vi "Queue Basics.vi"() -> ()   [LabVIEW 2012]
doc: "该范例演示了“获取队列引用”的使用方法，以及不同设置对队列操作的影响。通过队列在元素入队列（产生数据）和元素出队列（消费数据）之间传递数据。如两个循环的速度相同，队列将不会被填满。\n\n如元素入队列循环的速度大于元素出队列的速度，队列将被填满。元素入队列循环必须等待元素出队列循环移出队列中的元素。如元素入队列循环的速度小于元素出队列的速度，队列将被清空。元素出队列循环必须等待元素入队列循环填充队列中的元素。"
panel:
  out "Last Element Removed":dbl caption="最后删除的元素" format="%0.2f"
  in  "Enqueue Speed":bool caption="入队列速度"
  in  "Dequeue Speed":bool caption="出队列速度"
  out "Waveform Chart":cluster{"Last Element Inserted":dbl, dbl}(graph) caption="波形图表"
  out "Elements in Queue":i32(slide) caption="队列中的元素" scale=0.0..50.0 scale format="%0.0f"
  in  "stop":bool caption="停止"
  in  "Queue Size":i32=50 caption="队列大小"
  out "Last Element Inserted":dbl caption="最后插入的元素" format="%0.2f"
  # "操作步骤：\n1.设置要使用的队列大小。\n2.运行VI。\n3.调整“入队列速度”输入控件和“出队列速度”输入控件的值，查看队列显示控件中的元素和波形图表中曲线的改变。"
  # "最快(100ms)\n最慢(500ms)"
  # "最快(100ms)\n最慢(500ms)"
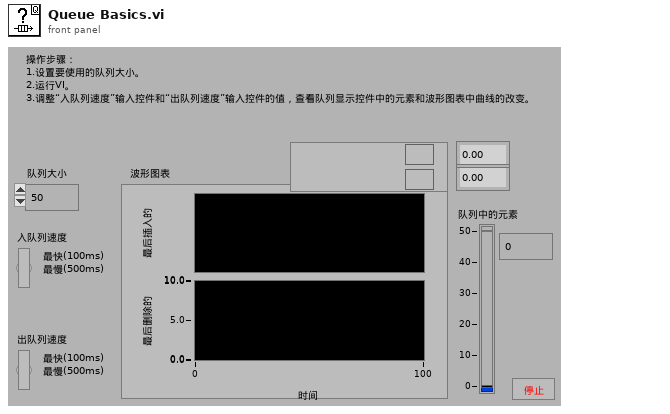
[diagram p1: front panel]
types:
  T1 = cluster{"Last Element Inserted":dbl, "Last Element Removed":dbl}
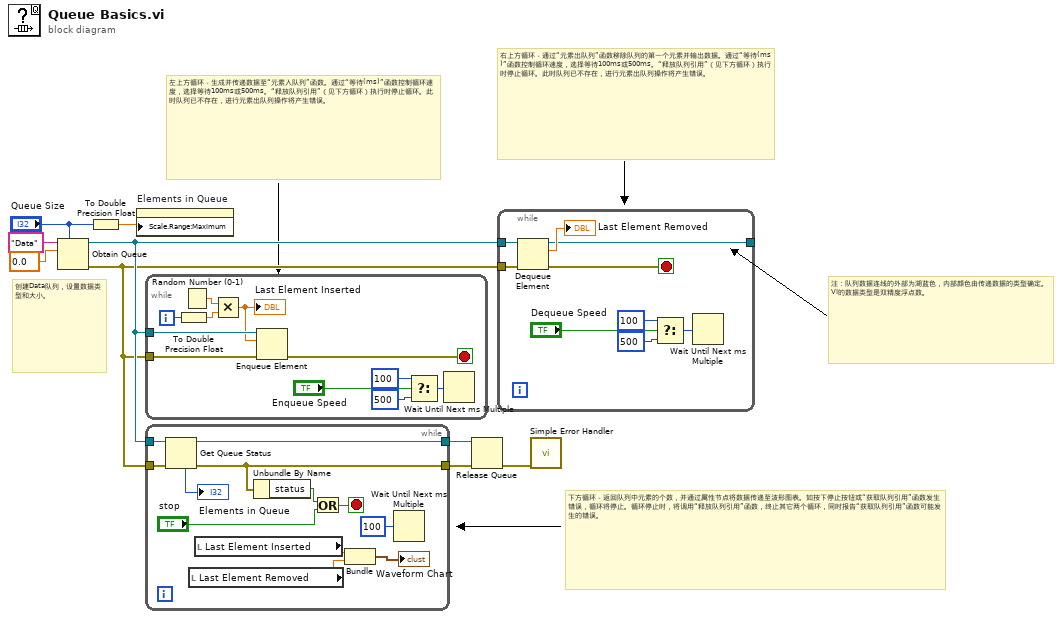
[diagram p0: block diagram]
diagram:
  # "右上方循环－通过“元素出队列”函数移除队列的第一个元素并输出数据。通过“等待(ms)”函数控制循环速度，选择等待100ms或500ms。“释放队列引用”（见下方循环）执行时停止循环。此时队列已不存在，进行元素出队列操作将产生错误。"
  # "注：队列数据连线的外部为湖蓝色，内部颜色由传递数据的类型确定。VI的数据类型是双精度浮点数。"
  # "下方循环－返回队列中元素的个数，并通过属性节点将数据传递至波形图表。如按下停止按钮或“获取队列引用”函数发生错误，循环将停止。循环停止时，将调用“释放队列引用”函数，终止其它两个循环，同时报告“获取队列引用”函数可能发生的错误。"
  # "左上方循环－生成并传递数据至“元素入队列”函数。通过“等待(ms)”函数控制循环速度，选择等待100ms或500ms。“释放队列引用”（见下方循环）执行时停止循环。此时队列已不存在，进行元素出队列操作将产生错误。"
  # "创建Data队列，设置数据类型和大小。"
  n1 = Obtain Queue(max queue size (-1, unlimited)="Queue Size", name (unnamed)="Data", element data type=0.0) -> (queue out=w9:refnum<queue>, error out=w4:errorcluster)  [unwired: 2 in, 1 out]
  n2 = To Double Precision Float(number="Queue Size") -> (double precision float=w8:dbl)
  n3 = property on="Elements in Queue" class="Slide (严格)"("Scale.Range:Maximum"=w8) -> ()  [unwired: 2 in, 2 out]
  n4 = while {
    tunnel: w9 -> [w20]
    tunnel: w4 -> [w11]
    i -> [w18]
    stop <- w10 stop-if-true
    n5 = To Double Precision Float(number=w18) -> (double precision float=w17:dbl)
    n6 = Random Number (0-1)() -> (number: 0 to 1=w19:dbl)
    n7 = Multiply(x=w19, y=w17) -> (x*y=w16:dbl)
    "Last Element Inserted" <- w16
    n8 = Enqueue Element(queue=w20, element=w16, error in (no error)=w11) -> (error out=w10:errorcluster)  [unwired: 3 out]
    n9 = Select(t=u32 100, s="Enqueue Speed", f=u32 500) -> (s? t:f=w12:u32)
    n10 = Wait Until Next ms Multiple(millisecond multiple=w12) -> ()  [unwired: 1 out]
  }
  n11 = while {
    tunnel: w9 -> [w32]
    tunnel: [w21] -> w3
    tunnel: w4 -> [w25]
    tunnel: [w22] -> w2
    stop <- w28 stop-if-true
    n12 = Get Queue Status(queue=w32, error in (no error)=w25) -> (queue out=w22:refnum<queue>, error out=w21:errorcluster, # elements in queue=→"Elements in Queue":i32)  [unwired: 6 out]
    n13 = local read "Last Element Removed"() -> (w23:dbl)
    n14 = local read "Last Element Inserted"() -> (w24:dbl)
    n15 = Unbundle By Name(w21) -> ("status"=w27:bool)
    n16 = Or(x=w27, y="stop") -> (x .or. y?=w28:bool)
    n17 = Bundle("Last Element Inserted"=w24, "Last Element Removed"=w23) -> (→"Waveform Chart":T1)  [unwired: 1 out]
    n18 = Wait Until Next ms Multiple(millisecond multiple=u32 100 ("milliseconds to wait")) -> ()  [unwired: 1 out]
  }
  n19 = Release Queue(queue=w2, error in (no error)=w3) -> (error out=w1:errorcluster)  [unwired: 3 out]
  n20 = while {
    tunnel: w9 -> [w41]
    tunnel: [w35] -> _
    tunnel: w4 -> [w34]
    stop <- w33 stop-if-true
    n21 = Dequeue Element(queue=w41, error in (no error)=w34) -> (queue out=w35:refnum<queue>, element=→"Last Element Removed":dbl, error out=w33:errorcluster)  [unwired: 2 out]
    n22 = Select(t=u32 100, s="Dequeue Speed", f=u32 500) -> (s? t:f=w37:u32)
    n23 = Wait Until Next ms Multiple(millisecond multiple=w37) -> ()  [unwired: 1 out]
  }
  n24 = call <vilib>:"Simple Error Handler.vi"("error in (no error)"=w1) -> ()  [unwired: 1 in, 8 out]
